vi "Internecine Avoider.vi"(7 "net address":u32, 8 "error in":errorcluster, 10 "service name":string, 11 "port":u16) -> (0 "error out":errorcluster, 3 "connection ID":refnum<k5>)   [LabVIEW 2020]
uses:
  <vilib>/Utility/tcp.llb/TCP Listen List Operations.ctl
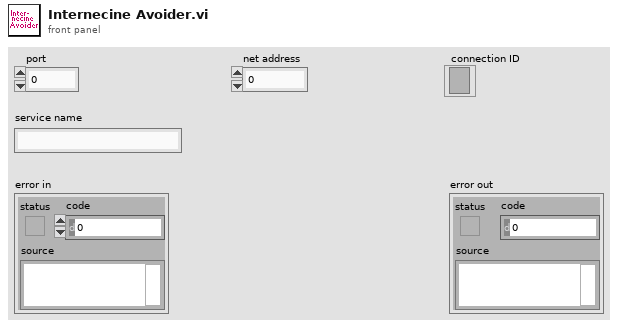
[diagram p1: front panel]
types:
  T1 = typedef "TCP Listen List Operations.ctl" = enum16{"Search", "Retrieve Element", "Add Element", "Delete Element"}
  T2 = cluster{"port":u16, "service name":string, "connection":refnum<k5>, "net address":u32}
  T3 = cluster{"port":u16, "service name":string, "listener ID":refnum<k5>, "net address":u32}
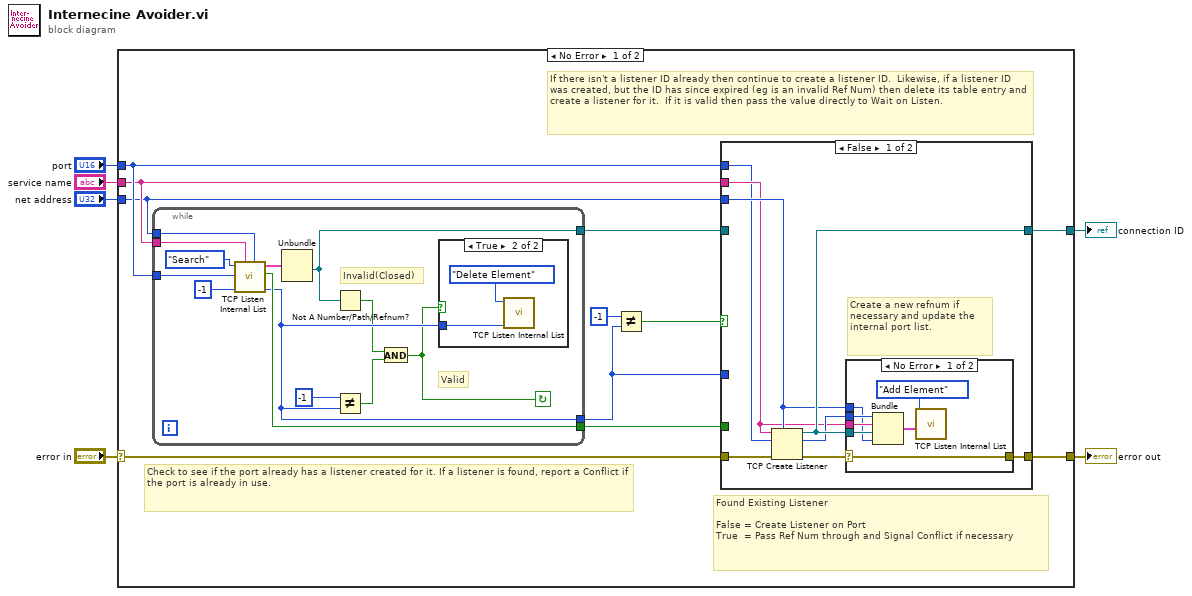
[diagram p0: block diagram]
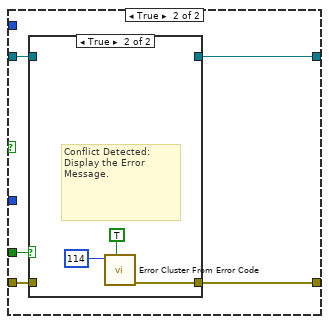
[diagram p4: hidden frame]
diagram:
  n1 = case shown="No Error" "error in" {
    selector: "error in" -> [w15 w59]
    tunnel: [w13 _] -> w6
    tunnel: [w11 w59] -> w5
    tunnel: "service name" -> [w8 _]
    tunnel: "net address" -> [w7 _]
    tunnel: "port" -> [w9 _]
    frame No Error {
      # "Check to see if the port already has a listener created for it. If a listener is found, report a Conflict if the port is already in use."
      # "If there isn't a listener ID already then continue to create a listener ID.  Likewise, if a listener ID was created, but the ID has since expired (eg is an invalid Ref Num) then delete its table entry and create a listener for it.  If it is valid then pass the value directly to Wait on Listen."
      # "Found Existing Listener\n\nFalse = Create Listener on Port\nTrue  = Pass Ref Num through and Signal Conflict if necessary"
      n2 = while {
        tunnel: [w24] -> w16
        tunnel: [w25] -> w14
        tunnel: [w27] -> w12
        tunnel: w9 -> [w26]
        tunnel: w8 -> [w19]
        tunnel: w7 -> [w18]
        stop <- w20 continue-if-true
        # "Valid"
        # "Invalid(Closed)"
        n3 = call <vilib>:"TCP Listen Internal List.vi"("net address"=w18, "service name"=w19, "Index #"=-1, "Port"=w26, "Operation"=TCP_Listen_List_Operations."Search") -> ("Element # \n(-1 if not found)"=w24:i32, "Conflict"=w27:bool, "Item Requested"=w28:T2)  [unwired: 1 in, 3 out]
        n4 = Unbundle(w28) -> ("connection"=w25:refnum<k5>)  [unwired: 3 out]
        n5 = Not A Number/Path/Refnum?(number/path/refnum=w25) -> (NaN/Path/Refnum?=w21:bool)
        n6 = Not Equal?(x=-1, y=w24) -> (x != y?=w22:bool)
        n7 = And(x=w21, y=w22) -> (x .and. y?=w20:bool)
        n8 = case shown="True" w20 {
          tunnel: w24 -> [_ w31]
          frame False {
          }
          frame True {
            n9 = call <vilib>:"TCP Listen Internal List.vi"("Index #"=w31, "Operation"=TCP_Listen_List_Operations."Delete Element") -> ()  [unwired: 4 in, 6 out]
          }
        }
      }
      n10 = Not Equal?(x=-1 ("y"), y=w16) -> (x != y?=w10:bool)
      n11 = case shown="False" w10 {
        tunnel: w16 -> [_ _]
        tunnel: w15 -> [w40 w53]
        tunnel: [w39 w49] -> w13
        tunnel: [w38 w52] -> w11
        tunnel: w14 -> [_ w50]
        tunnel: w12 -> [_ w51]
        tunnel: w9 -> [w33 _]
        tunnel: w8 -> [w34 _]
        tunnel: w7 -> [w35 _]
        frame False {
          # "Create a new refnum if necessary and update the internal port list."
          n12 = TCP Create Listener(7:w35, 8:w40, 10:w33, 11:w34) -> (0:w36:errorcluster, 2:w37:u16, 3:w39:refnum<k5>)  [unwired: 1 out]
          n13 = case shown="No Error" w36 {
            selector: w36 -> [w44 w48]
            tunnel: w37 -> [w47 _]
            tunnel: w39 -> [w45 _]
            tunnel: [w44 w48] -> w38
            tunnel: w34 -> [w42 _]
            tunnel: w35 -> [w41 _]
            frame No Error {
              n14 = Bundle("port"=w47, "service name"=w42, "listener ID"=w45, "net address"=w41) -> (w43:T3)  [unwired: 1 out]
              n15 = call <vilib>:"TCP Listen Internal List.vi"("Element In"=w43, "Operation"=TCP_Listen_List_Operations."Add Element") -> ()  [unwired: 4 in, 6 out]
            }
            frame Error {
            }
          }
        }
        frame True {
          n16 = case shown="True" w51 {
            tunnel: w53 -> [w55 _]
            tunnel: [w55 w57] -> w52
            tunnel: w50 -> [w54 _]
            tunnel: [w54 _] -> w49
            frame False {
              # "No Conflict. Refnum can be reused, just pass it through."
            }
            frame True {
              # "Conflict Detected: Display the Error Message."
              n17 = call <vilib>:"Error Cluster From Error Code.vi"("show call chain? (False)"=TRUE, "error code (0)"=114 ("error code (114)")) -> ("error out"=w57:errorcluster)  [unwired: 7 in]
            }
          }
        }
      }
    }
    frame Error {
    }
  }
  "error out" <- w5
  "connection ID" <- w6
